vi "ZDataVIS_Parse_AO+Lockin_Config.vi"(10 "Only Read 1st YAML":bool, 11 "\"notes \"":string[](array[string])) -> (1 "wirings":string[][][](array[string]), 2 "wiring":string[][](array[string]), 3 "all lockin AO":T1[](array[typedef]) {"AO f (Hz)" min=0.001 max=10000.0; "AO DC (V)" format="%.3p"; "AO Amp (V)" format="%.3p"})   [LabVIEW 2016]
uses:
  <userlib>/LevyLab/Lockin-Multichannel/Instrument.Lockin/Typedefs/AO-cluster.ctl
  <userlib>/LevyLab/Lockin-Multichannel/Instrument.Lockin/Typedefs/AO_Amp-array.ctl
  <userlib>/LevyLab/Lockin-Multichannel/Instrument.Lockin/Typedefs/AO_DC-array.ctl
  <userlib>/LevyLab/Lockin-Multichannel/Instrument.Lockin/Typedefs/AO_f-array.ctl
  <userlib>/LevyLab/Lockin-Multichannel/Instrument.Lockin/Typedefs/AO_phi-array.ctl
  <userlib>/LevyLab/Lockin-Multichannel/Instrument.Lockin/Typedefs/Function-array.ctl
  <userlib>/LevyLab/Lockin-Multichannel/Instrument.Lockin/Typedefs/Function-enum.ctl
  <vilib>/addons/WireFlow/_WF_ProgressBar.llb/ProgressBar_WireFlow.lvclass
  <vilib>/addons/WireFlow/_WF_ProgressBar.llb/MessageTextType.ctl
  <vilib>/MakerHub/Toolbox/LMH-Toolbox.lvlib
  <userlib>/LevyLab/Lockin-Multichannel/Instrument.Lockin/Instrument.Lockin.lvclass
panel:
  out "WF-ProgressBar out":refnum<class "ProgressBar_WireFlow.lvclass">
  out "F":dbl[](array[numeric])
  out "AC":dbl[](array[numeric])
  out "DC":dbl[](array[numeric])
  out "lockin contents":string[][](array[string])
  # "1"
  # "2"
  # "3"
  # "4"
  # "5"
  # "6"
  # "7"
  # "8"
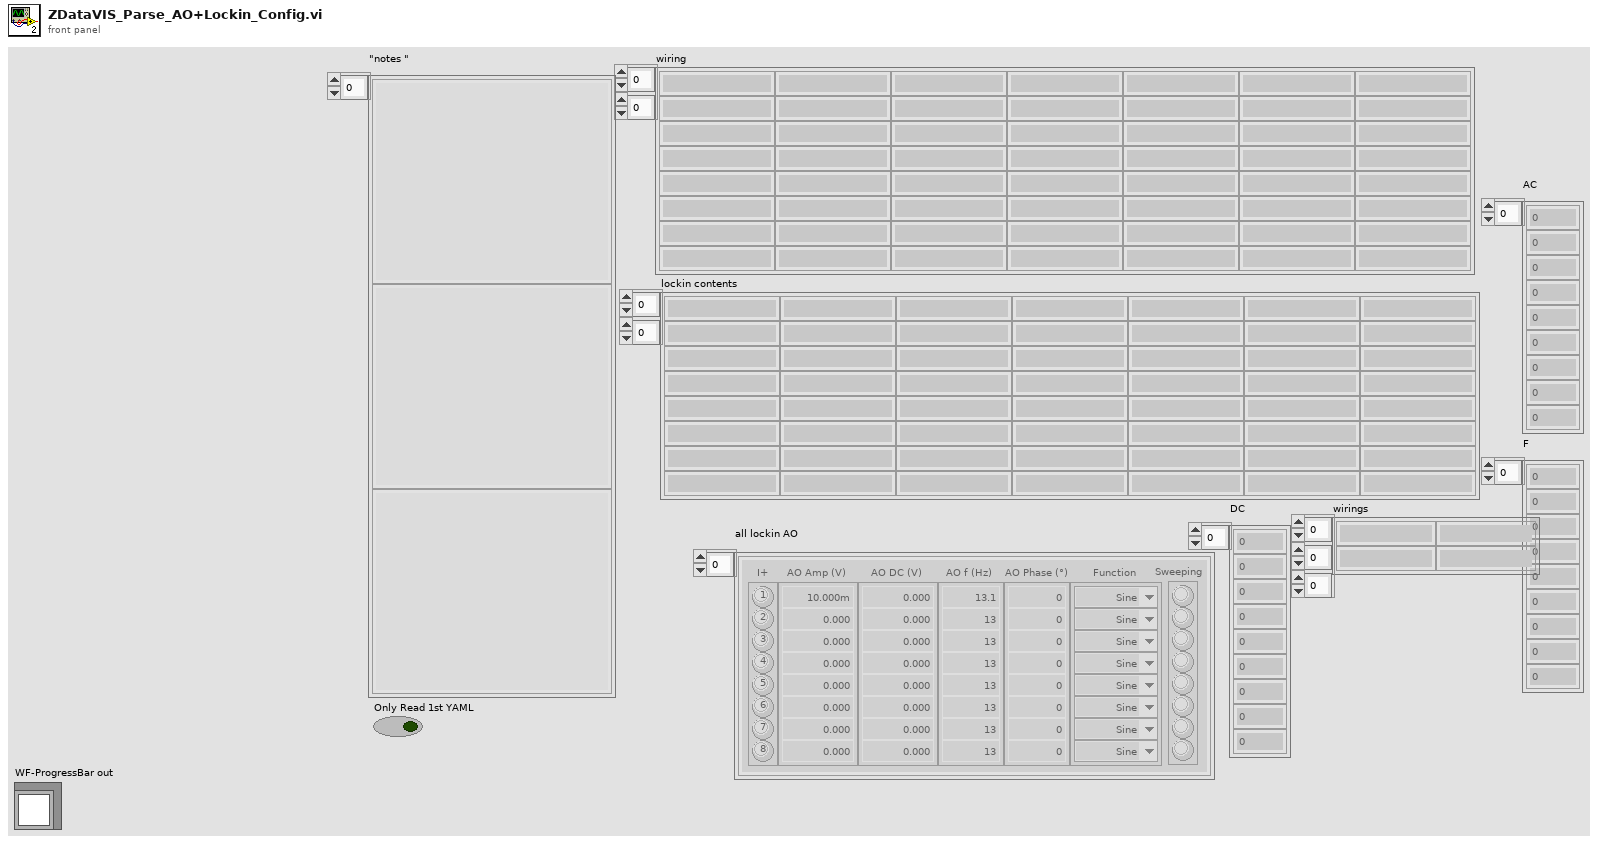
[diagram p1: front panel]
types:
  T1 = typedef "Instrument.Lockin.lvclass/AO-cluster.ctl" = cluster{"AO Amp (V)":T2, "AO DC (V)":T3, "AO f (Hz)":T4, "AO Phase (°)":T5, "Function":T6, "I+":bool[], "Sweeping":bool[]}
  T2 = typedef "Instrument.Lockin.lvclass/AO_Amp-array.ctl" = dbl[]
  T3 = typedef "Instrument.Lockin.lvclass/AO_DC-array.ctl" = dbl[]
  T4 = typedef "Instrument.Lockin.lvclass/AO_f-array.ctl" = dbl[]
  T5 = typedef "Instrument.Lockin.lvclass/AO_phi-array.ctl" = dbl[]
  T6 = typedef "Instrument.Lockin.lvclass/Function-array.ctl" = T7[]
  T7 = typedef "Instrument.Lockin.lvclass/Function-enum.ctl" = enum16{"Sine", "Triangle", "Square", "Sawtooth"}
  T8 = typedef "ProgressBar_WireFlow.lvclass/MessageTextType.ctl" = enum16{"Title", "General", "Current item"}
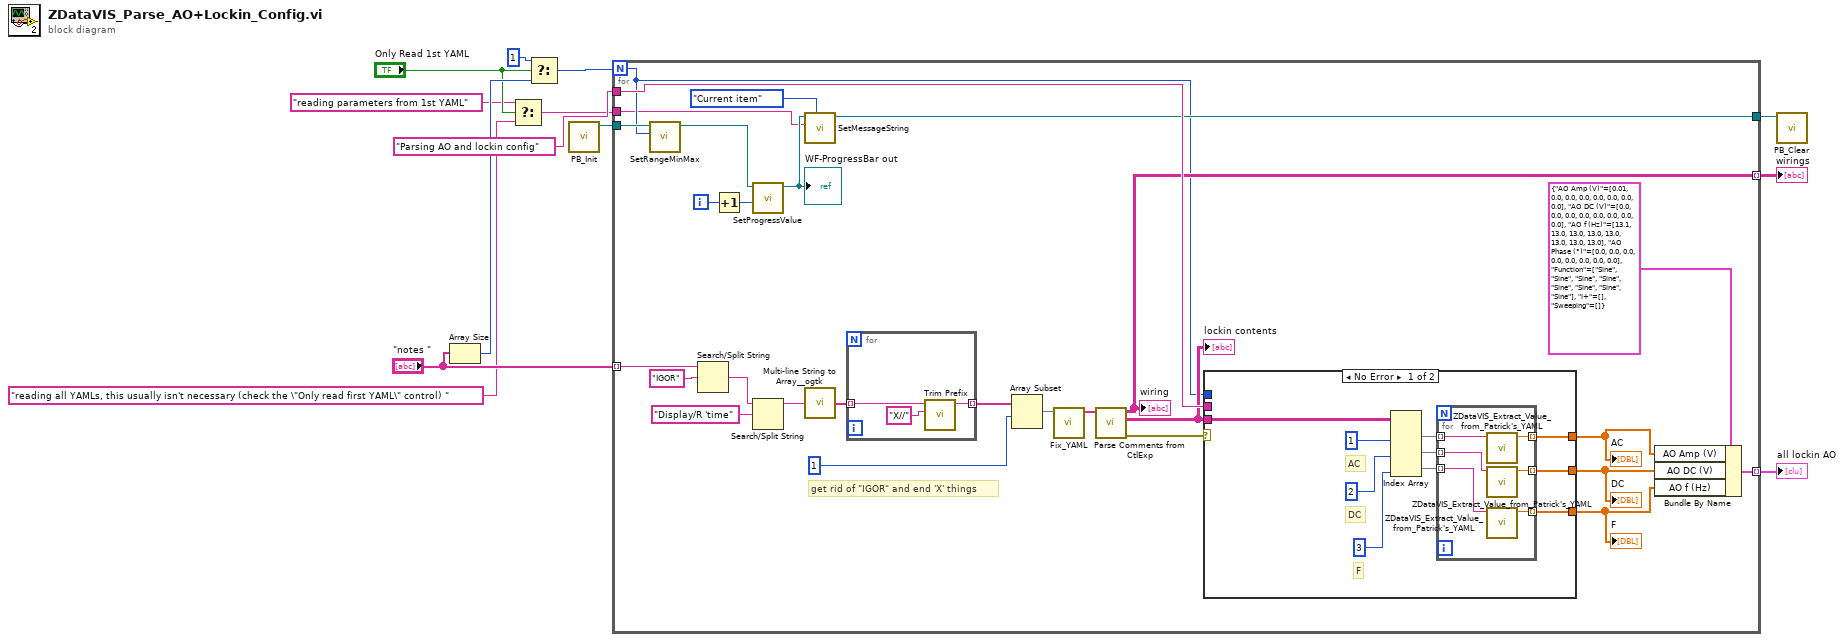
[diagram p0: block diagram]
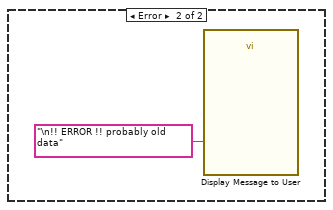
[diagram p2: hidden frame]
diagram:
  n1 = Array Size(array="\"notes \"") -> (size(s)=w8:i32)
  n2 = Select(t="reading parameters from 1st YAML" ("f"), s="Only Read 1st YAML", f="reading all YAMLs, this usually isn't necessary (check the \"Only read first YAML\" control) ") -> (s? t:f=w3:string)
  n3 = Select(t=1, s="Only Read 1st YAML", f=w8) -> (s? t:f=w11:i32)
  n4 = call <vilib>:"PB_Init.vi"() -> ("WF-ProgressBar out"=w5:refnum<class "ProgressBar_WireFlow.lvclass">)  [unwired: 10 in, 1 out]
  n5 = for {
    N: w11 -> [w17]
    tunnel: "\"notes \"" -> [w32] mode=indexing
    tunnel: [w30] -> w13 mode=indexing
    tunnel: "Parsing AO and lockin config" ("title (\"Progress\")") -> [w25]
    tunnel: [w24] -> w7 mode=indexing
    tunnel: [w22] -> w6
    tunnel: w5 -> [w20]
    tunnel: w3 -> [w14]
    i -> [w16]
    # "get rid of \"IGOR\" and end 'X' things"
    n6 = call-dynamic "SetRangeMinMax.vi"("Max (1)"=w17, "WF-ProgressBar in"=w20) -> ("WF-ProgressBar out"=w18:refnum<class "ProgressBar_WireFlow.lvclass">)  [unwired: 8 in, 1 out]
    n7 = Search/Split String(string=w32, search string/char (-)="IGOR") -> (match + rest of string=w40:string)  [unwired: 1 in, 2 out]
    n8 = Increment(x=w16) -> (x+1=w15:i32)
    n9 = call-dynamic "SetProgressValue.vi"("Value"=w15, "WF-ProgressBar in"=w18) -> ("WF-ProgressBar out"=w21:refnum<class "ProgressBar_WireFlow.lvclass">)  [unwired: 7 in, 2 out]
    "WF-ProgressBar out" <- w21
    n10 = Search/Split String(string=w40, search string/char (-)="Display/R 'time") -> (substring before match=w38:string)  [unwired: 1 in, 2 out]
    n11 = call-dynamic "SetMessageString.vi"("message field"=MessageTextType."Current item", "Message"=w14, "WF-ProgressBar in"=w21) -> ("WF-ProgressBar out"=w22:refnum<class "ProgressBar_WireFlow.lvclass">)  [unwired: 7 in, 1 out]
    n12 = call <userlib>:"Multi-line String to Array__ogtk.vi"("string"=w38) -> ("lines"=w37:string[])
    n13 = for {
      tunnel: w37 -> [w61] mode=indexing
      tunnel: [w59] -> w35 mode=indexing
      n14 = call <vilib>:"Trim Prefix.vi"("Prefix"="X//", "String"=w61) -> ("String"=w59:string)  [unwired: 9 in]
    }
    n15 = Array Subset(array=w35, index=1) -> (w34:string[])  [unwired: 1 in]
    n16 = call "Fix_YAML.vi"("Array in"=w34) -> ("Array out"=w33:string[])  [unwired: 10 in]
    n17 = call "Parse Comments from CtlExp.vi"("ENTIRE Array of YAML Lines"=w33) -> ("error out"=w26:errorcluster, "lockin contents"=w23:string[][], "wiring"=w24:string[][])  [unwired: 6 in, 1 out]
    "wiring" <- w24
    "lockin contents" <- w23
    n18 = case shown="No Error" w26 {
      tunnel: w23 -> [w51 _]
      tunnel: [w44 _] -> w29
      tunnel: [w43 _] -> w28
      tunnel: [w42 _] -> w27
      tunnel: w17 -> [_ _]
      tunnel: w25 -> [_ _]
      frame No Error {
        # "F"
        # "DC"
        # "AC"
        n19 = Index Array(array=w51, index (col) #1=1 ("disabled index (col)"), index (col) #2=2 ("index (col)"), index (col) #3=3 ("index (col)")) -> (element #1=w49:string[], element #2=w48:string[], element #3=w45:string[])  [unwired: 3 in]
        n20 = for {
          tunnel: w49 -> [w57] mode=indexing
          tunnel: w48 -> [w54] mode=indexing
          tunnel: [w55] -> w43 mode=indexing
          tunnel: [w56] -> w44 mode=indexing
          tunnel: w45 -> [w53] mode=indexing
          tunnel: [w52] -> w42 mode=indexing
          n21 = call "ZDataVIS_Extract_Value_from_Patrick's_YAML.vi"("String"=w57) -> ("Numeric"=w56:dbl)  [unwired: 10 in]
          n22 = call "ZDataVIS_Extract_Value_from_Patrick's_YAML.vi"("String"=w54) -> ("Numeric"=w55:dbl)  [unwired: 10 in]
          n23 = call "ZDataVIS_Extract_Value_from_Patrick's_YAML.vi"("String"=w53) -> ("Numeric"=w52:dbl)  [unwired: 10 in]
        }
      }
      frame Error {
        n24 = call "Display Message to User"("Message"="\n!! ERROR !! probably old data" ("string")) -> ()  [unwired: 9 in, 2 out]
      }
    }
    "DC" <- w28
    "AC" <- w29
    "F" <- w27
    n25 = Bundle By Name(cluster=T1 {"AO Amp (V)"=[0.01, 0.0, 0.0, 0.0, 0.0, 0.0, 0.0, 0.0], "AO DC (V)"=[0.0, 0.0, 0.0, 0.0, 0.0, 0.0, 0.0, 0.0], "AO f (Hz)"=[13.1, 13.0, 13.0, 13.0, 13.0, 13.0, 13.0, 13.0], "AO Phase (°)"=[0.0, 0.0, 0.0, 0.0, 0.0, 0.0, 0.0, 0.0], "Function"=[enum."Sine", enum."Sine", enum."Sine", enum."Sine", enum."Sine", enum."Sine", enum."Sine", enum."Sine"], "I+"=[], "Sweeping"=[]} ("Channels: AO"), "AO Amp (V)"=w29, "AO DC (V)"=w28, "AO f (Hz)"=w27) -> (w30:T1)
  }
  "all lockin AO" <- w13
  "wirings" <- w7
  n26 = call-dynamic "PB_Clear.vi"("WF-ProgressBar in"=w6) -> ()  [unwired: 9 in, 2 out]
